vi "read timing status tags.vi"(8 "error in":errorcluster, 11 "Standard Engine Configuration in":refnum<class "Standard Engine Configuration.lvclass">) -> (0 "error out":errorcluster, 2 "timing reporting":T1, 3 "Standard Engine Configuration out":refnum<class "Standard Engine Configuration.lvclass">)   [LabVIEW 2013, in "Standard Engine Configuration.lvclass"]
uses:
  Standard Engine Configuration.lvclass
  timing reporting tags.ctl
  Standard Engine Configuration.lvclass/Standard Engine Configuration.ctl
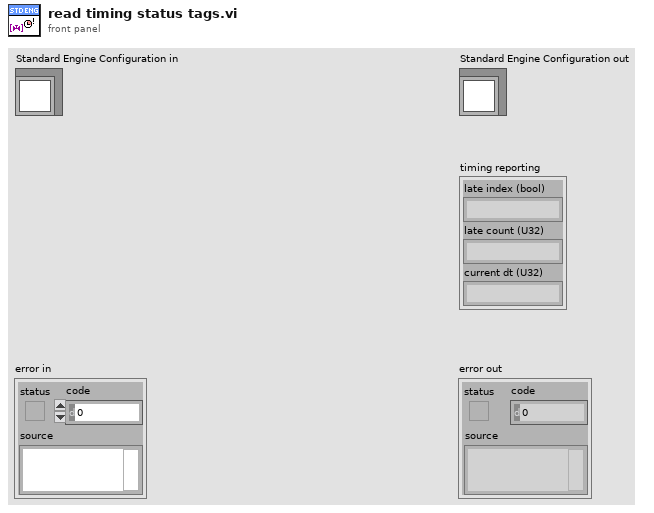
[diagram p1: front panel]
types:
  T1 = typedef "Standard Engine Configuration.lvclass/timing reporting tags.ctl" = cluster{"late index (bool)":string, "late count (U32)":string, "current dt (U32)":string}
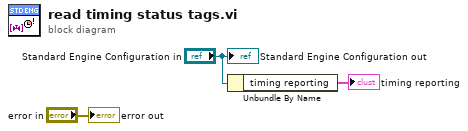
[diagram p0: block diagram]
diagram:
  n1 = Unbundle By Name("Standard Engine Configuration in") -> ("timing reporting"=→"timing reporting":T1)
  "error out" <- "error in"
  "Standard Engine Configuration out" <- "Standard Engine Configuration in"
